vi "Translator.File.Read.Flag.vi"(8 "error in":errorcluster, 9 "miniature (F)":bool, 10 "Language in use":string="English", 11 "Translation file":path=path "D:/PL_0125_Sapphire_Automation_branches/SOFTWARE_v1.1-Translation/settings/Translation-Chinese.ini") -> (0 "error out":errorcluster, 1 "~flag small":picture, 2 "~flag":picture)   [LabVIEW 2016]
uses:
  <vilib>/Utility/miscctls.llb/LVBoundsTypeDef.ctl
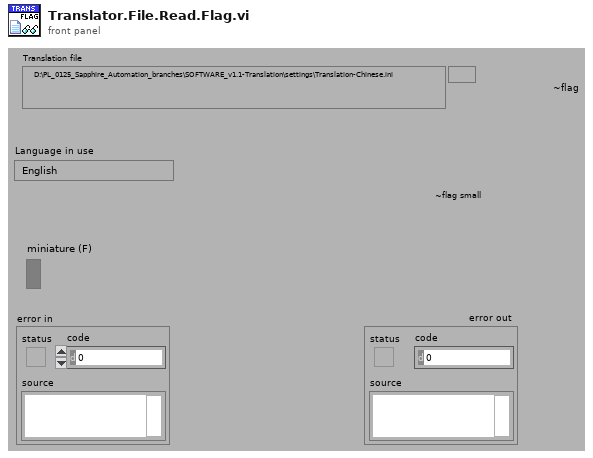
[diagram p1: front panel]
types:
  T1 = typedef "LVBoundsTypeDef.ctl" = cluster{"Width":u32, "Height":u32}
  T2 = typedef "imagedata.ctl" = cluster{"image type":i32, "image depth":i32, "image":u8[], "mask":u8[], "colors":u32[], "Rectangle":cluster{"left":i16, "top":i16, "right":i16, "bottom":i16}}
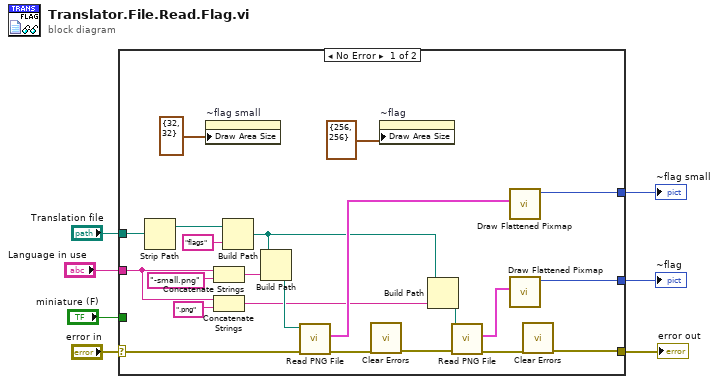
[diagram p0: block diagram]
diagram:
  n1 = case shown="No Error" "error in" {
    selector: "error in" -> [w28 w30]
    tunnel: [w18 w30] -> w7
    tunnel: "Translation file" -> [w22 _]
    tunnel: "Language in use" -> [w12 _]
    tunnel: [w26 _] -> w3
    tunnel: "miniature (F)" -> [_ _]
    tunnel: [w17 _] -> w1
    frame No Error {
      n2 = Strip Path(path=w22) -> (stripped path=w24:path)  [unwired: 1 out]
      n3 = property on="~flag small" class="Pict"("Draw Area Size"=T1 {"Width"=32, "Height"=32}) -> ()  [unwired: 2 in, 2 out]
      n4 = Concatenate Strings(w12, "-small.png" ("string")) -> (w29:string)
      n5 = Concatenate Strings(w12, ".png" ("string")) -> (w10:string)
      n6 = Build Path(base path=w24, name or relative path="flags") -> (appended path=w15:path)
      n7 = Build Path(base path=w15, name or relative path=w29) -> (appended path=w27:path)
      n8 = call <vilib>:"Read PNG File.vi"("error in (no error)"=w28, "path to PNG file"=w27) -> ("error out"=w21:errorcluster, "image data"=w25:T2)  [unwired: 7 in, 1 out]
      n9 = call <vilib>:"Clear Errors.vi"("error in (no error)"=w21) -> ("error out"=w20:errorcluster)  [unwired: 5 in, 1 out]
      n10 = property on="~flag" class="Pict"("Draw Area Size"=T1 {"Width"=256, "Height"=256}) -> ()  [unwired: 2 in, 2 out]
      n11 = Build Path(base path=w15, name or relative path=w10) -> (appended path=w14:path)
      n12 = call <vilib>:"Read PNG File.vi"("error in (no error)"=w20, "path to PNG file"=w14) -> ("error out"=w19:errorcluster, "image data"=w16:T2)  [unwired: 7 in, 1 out]
      n13 = call <vilib>:"Draw Flattened Pixmap.vi"("image data"=w25) -> ("new picture"=w26:picture)  [unwired: 8 in]
      n14 = call <vilib>:"Draw Flattened Pixmap.vi"("image data"=w16) -> ("new picture"=w17:picture)  [unwired: 8 in]
      n15 = call <vilib>:"Clear Errors.vi"("error in (no error)"=w19) -> ("error out"=w18:errorcluster)  [unwired: 5 in, 1 out]
    }
    frame Error {
    }
  }
  "error out" <- w7
  "~flag small" <- w3
  "~flag" <- w1
